vi "Dimmer Get Value From BaseStation.vi"() -> ()   [LabVIEW 2014, in "ESP8266 WiFi Wrapper.lvlib"]
uses:
  ESP8266 WiFi Wrapper.lvlib
  <vilib>/Aledyne-TSXperts/Arduino Compatible Compiler for LabVIEW/Arduino Compatible Compiler for LabVIEW.lvlib
panel:
  out "Bytes read":i16
  in  "Connect to IP":u8[](array[numeric])=[192, 168, 0, 42]
  in  "DNS":u8[](array[numeric])=[0, 0, 0, 0]
  in  "IP address":u8[](array[numeric])=[192, 168, 0, 47]
  in  "Gateway":u8[](array[numeric])=[192, 168, 0, 1]
  in  "Subnet mask":u8[](array[numeric])=[255, 255, 255, 0]
  in  "Password":string="12345678"
  in  "SSID":string="ESP8266 Wifi Example"
  in  "error in (no error)":errorcluster
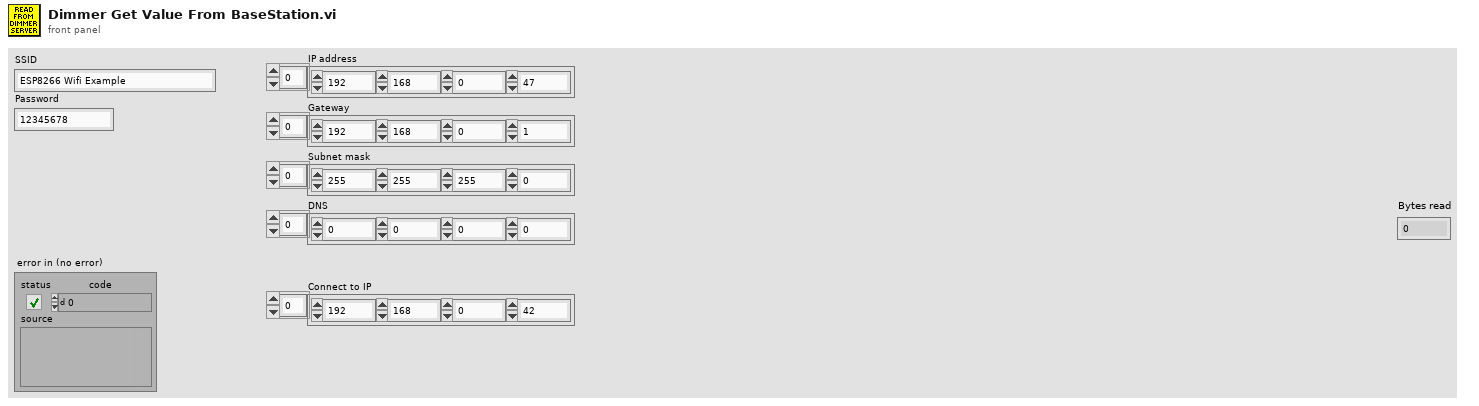
[diagram p1: front panel]
types:
  T1 = enum16{"WIFI_OFF", "WIFI_STA", "WIFI_AP", "WIFI_AP_STA"}
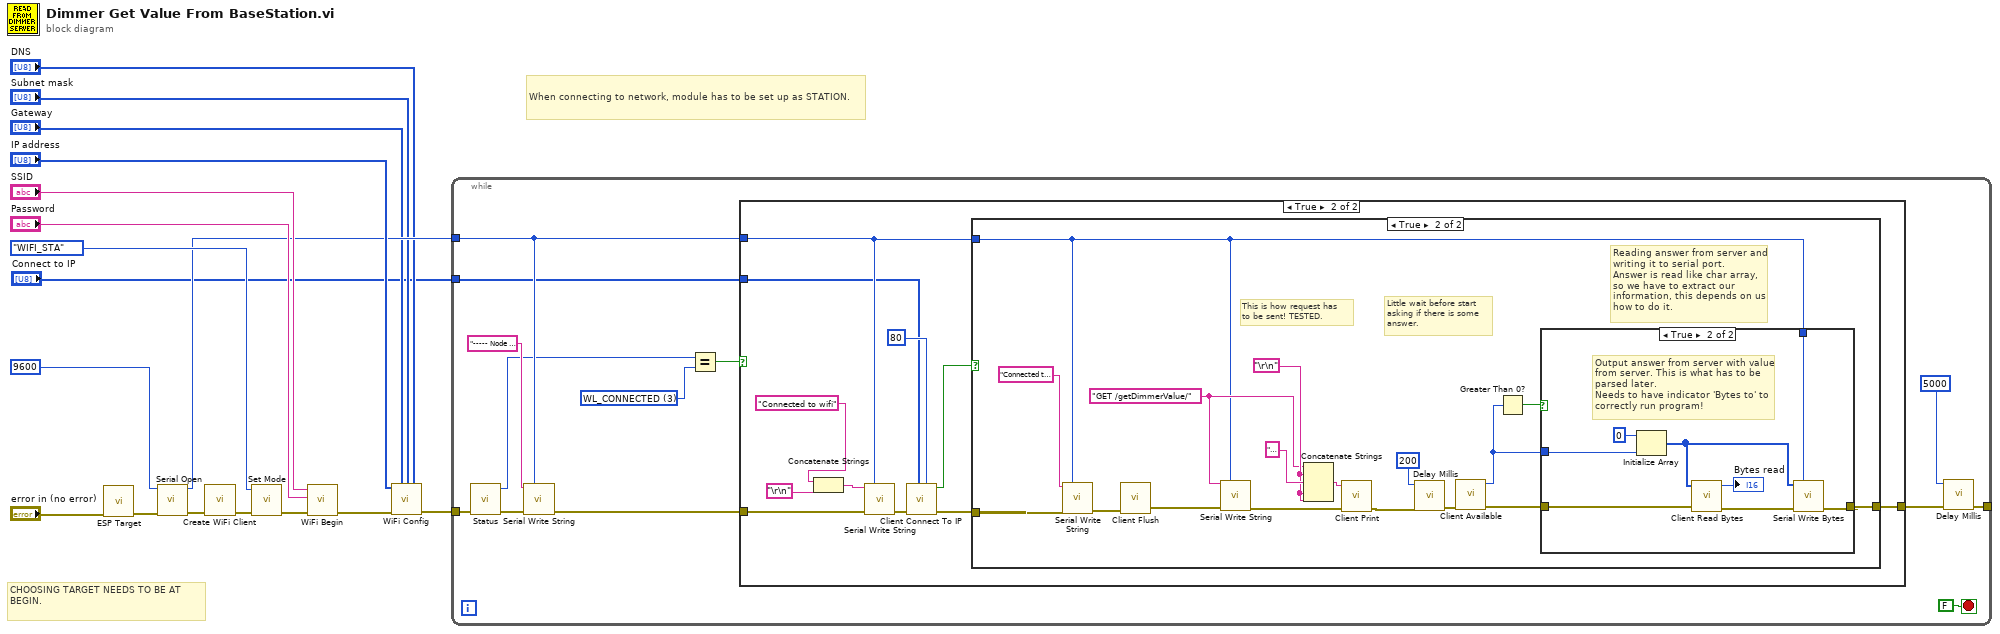
[diagram p0: block diagram]
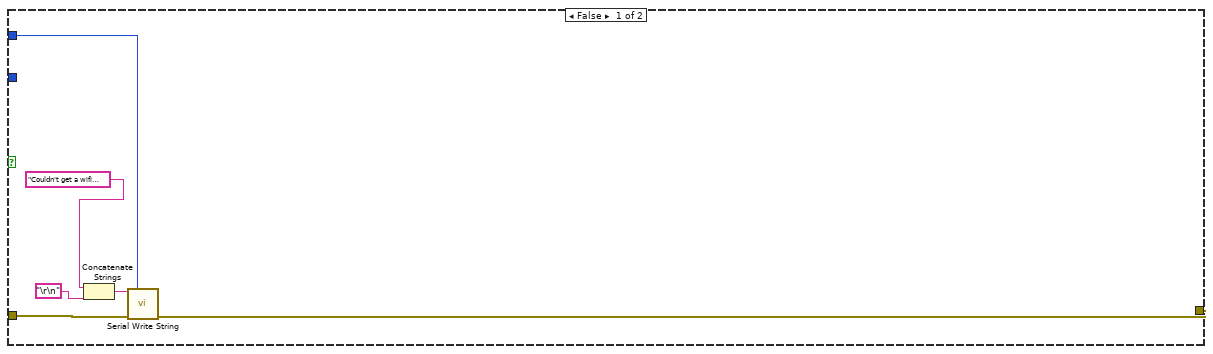
[diagram p2: hidden frame]
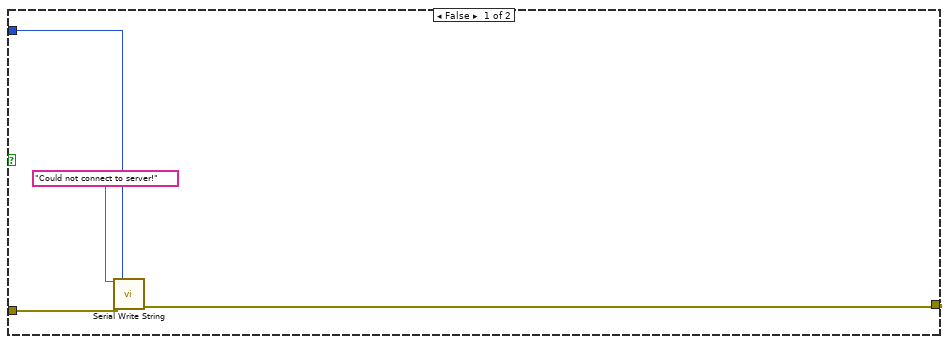
[diagram p3: hidden frame]
diagram:
  # "CHOOSING TARGET NEEDS TO BE AT BEGIN."
  # "When connecting to network, module has to be set up as STATION."
  n1 = call "ESP Target.vi"("Error In"="error in (no error)") -> ("Error Out"=w3:errorcluster)  [unwired: 10 in]
  n2 = call <vilib>:"Serial Open.vi"("Speed"=u32 9600, "error in (no error)"=w3) -> ("Instance"=w10:u8, "error out"=w9:errorcluster)  [unwired: 12 in]
  n3 = call "Create WiFi Client.vi"("Error In"=w9) -> ("Error Out"=w1:errorcluster)  [unwired: 10 in]
  n4 = call "Set Mode.vi"("Error In"=w1, "WiFi Server Mode"=T1."WIFI_STA") -> ("Error Out"=w13:errorcluster)  [unwired: 9 in]
  n5 = call "WiFi Begin.vi"("Error In"=w13, "Password"="Password", "SSID"="SSID") -> ("Error Out"=w11:errorcluster)  [unwired: 8 in]
  n6 = call "WiFi Config.vi"("IP address"="IP address", "Gateway address"="Gateway", "Subnet mask"="Subnet mask", "DNS address"="DNS", "Error In"=w11) -> ("Error Out"=w8:errorcluster)  [unwired: 10 in]
  n7 = while {
    tunnel: w10 -> [w25]
    tunnel: w8 -> [w29]
    tunnel: [w19] -> _
    tunnel: "Connect to IP" -> [w18]
    stop <- FALSE stop-if-true
    w23 = u8 3 items=["WL_NO_SHIELD"=255, "WL_IDLE_STATUS"=0, "WL_NO_SSID_AVAIL"=1, "WL_SCAN_COMPLETED"=2, "WL_CONNECTED"=3, "WL_CONNECT_FAILED"=4, "WL_CONNECTION_LOST"=5, "WL_DISCONNECTED"=6] ("Ring")
    n8 = call "Status.vi"("Error In"=w29) -> ("Error Out"=w27:errorcluster, "Status"=w22:u8)  [unwired: 9 in]
    n9 = call <vilib>:"Serial Write String.vi"("String"="----- Node 1 --------", "Instance"=w25, "error in (no error)"=w27) -> ("error out"=w26:errorcluster)  [unwired: 12 in]
    n10 = Equal?(x=w22, y=w23) -> (x = y?=w24:bool)
    n11 = case shown="True" w24 {
      tunnel: [w31 w38] -> w20
      tunnel: w25 -> [w36 w46]
      tunnel: w26 -> [w35 w47]
      tunnel: w18 -> [_ w37]
      frame False {
        n12 = Concatenate Strings("Couldn't get a wifi connection" ("String"), "\r\n" ("End of Line Constant")) -> (w32:string)
        n13 = call <vilib>:"Serial Write String.vi"("String"=w32, "Instance"=w36, "error in (no error)"=w35) -> ("error out"=w31:errorcluster)  [unwired: 12 in]
      }
      frame True {
        n14 = Concatenate Strings("Connected to wifi" ("String"), "\r\n" ("End of Line Constant")) -> (w41:string)
        n15 = call <vilib>:"Serial Write String.vi"("String"=w41, "Instance"=w46, "error in (no error)"=w47) -> ("error out"=w45:errorcluster)  [unwired: 12 in]
        n16 = call "Client Connect To IP.vi"("Port"=u32 80, "IP address"=w37, "Error In"=w45) -> ("Error Out"=w43:errorcluster, "Connected?"=w42:bool)  [unwired: 7 in]
        n17 = case shown="True" w42 {
          tunnel: w46 -> [w48 w53]
          tunnel: [w49 w66] -> w38
          tunnel: w43 -> [w50 w67]
          frame False {
            n18 = call <vilib>:"Serial Write String.vi"("String"="Could not connect to server!", "Instance"=w48, "error in (no error)"=w50) -> ("error out"=w49:errorcluster)  [unwired: 12 in]
          }
          frame True {
            w54 = "GET /getDimmerValue/" ("string")
            w57 = "\r\n" ("End of Line Constant")
            # "Little wait before start\nasking if there is some\nanswer."
            # "This is how request has\nto be sent! TESTED."
            # "Reading answer from server and\nwriting it to serial port.\nAnswer is read like char array,\nso we have to extract our\ninformation, this depends on us\nhow to do it."
            n19 = call <vilib>:"Serial Write String.vi"("String"="Connected to server.", "Instance"=w53, "error in (no error)"=w67) -> ("error out"=w60:errorcluster)  [unwired: 12 in]
            n20 = call "Client Flush.vi"("Error In"=w60) -> ("Error Out"=w55:errorcluster)  [unwired: 10 in]
            n21 = call <vilib>:"Serial Write String.vi"("String"=w54, "Instance"=w53, "error in (no error)"=w55) -> ("error out"=w56:errorcluster)  [unwired: 12 in]
            n22 = Concatenate Strings(w54, w57, "Connection: close" ("Input String"), w57, w57) -> (w59:string)
            n23 = call "Client Print.vi"("Error In"=w56, "Input String"=w59) -> ("Error Out"=w64:errorcluster)  [unwired: 9 in]
            n24 = call <vilib>:"Delay Millis.vi"("error in (no error)"=w64, "delay"=u32 200) -> ("error out"=w63:errorcluster)  [unwired: 9 in]
            n25 = call "Client Available.vi"("Error In"=w63) -> ("Error Out"=w62:errorcluster, "Chars to read"=w52:i16)  [unwired: 9 in]
            n26 = Greater Than 0?(x=w52) -> (x > 0?=w61:bool)
            n27 = case shown="True" w61 {
              tunnel: [w69 w76] -> w66
              tunnel: w53 -> [_ w77]
              tunnel: w62 -> [w69 w71]
              tunnel: w52 -> [_ w70]
              frame False {
              }
              frame True {
                # "Output answer from server with value\nfrom server. This is what has to be\nparsed later.\nNeeds to have indicator 'Bytes to' to\ncorrectly run program!"
                n28 = Initialize Array(u8 0, w70) -> (w73:u8[])
                n29 = call "Client Read Bytes.vi"("Error In"=w71, "Buffer"=w73) -> ("Error Out"=w72:errorcluster, "Bytes read"=→"Bytes read":i16)  [unwired: 8 in]
                n30 = call <vilib>:"Serial Write Bytes.vi"("Data"=w73, "Instance"=w77, "error in (no error)"=w72) -> ("error out"=w76:errorcluster)  [unwired: 12 in]
              }
            }
          }
        }
      }
    }
    n31 = call <vilib>:"Delay Millis.vi"("error in (no error)"=w20, "delay"=u32 5000) -> ("error out"=w19:errorcluster)  [unwired: 9 in]
  }
